vi "FgState.vi"(7 "Set (F)":bool, 11 "State In":string) -> (3 "State Out":string)   [LabVIEW 2018, in "ScopeModule.lvlib"]
uses:
  ScopeModule.lvlib
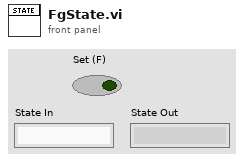
[diagram p1: front panel]
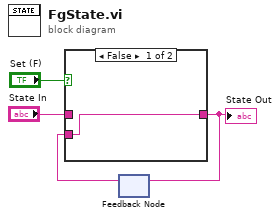
[diagram p0: block diagram]
diagram:
  n1 = feedback #1() -> (w1:string)  [unwired: 1 in]
  n2 = case shown="False" "Set (F)" {
    tunnel: "State In" -> [_ w6]
    tunnel: [w5 w6] -> w2
    tunnel: w1 -> [w5 _]
    frame False {
    }
    frame True {
    }
  }
  "State Out" <- w2
  n3 = feedback-in #1(w2) -> ()
